vi "Ctrl.StyleFont.vi"(8 "error in (no error)":errorcluster, 10 "Font Info":T1, 11 "Ctl Ref in":refnum<vi>) -> (0 "error out":errorcluster, 3 "Ctl Ref out":refnum<vi>)   [LabVIEW 2017, in "JKI Simple Localization.lvlib"]
uses:
  API/JKI Simple Localization.lvlib
  Definitions/Private/Font Info -- Cluster.ctl
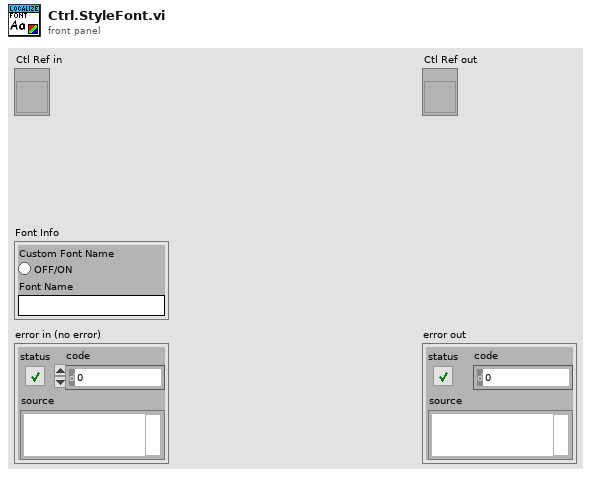
[diagram p1: front panel]
types:
  T1 = typedef "JKI Simple Localization.lvlib/Font Info -- Cluster.ctl" = cluster{"Custom Font Name":bool, "Font Name":string}
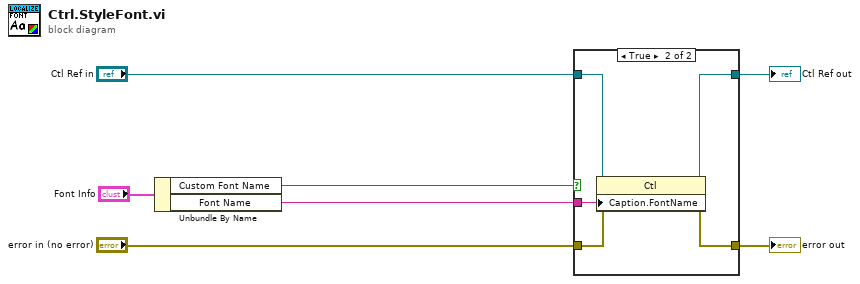
[diagram p0: block diagram]
diagram:
  n1 = Unbundle By Name("Font Info") -> ("Custom Font Name"=w4:bool, "Font Name"=w5:string)
  n2 = case shown="True" w4 {
    tunnel: "error in (no error)" -> [w8 w14]
    tunnel: [w9 w12] -> w2
    tunnel: "Ctl Ref in" -> [w9 w13]
    tunnel: w5 -> [_ w11]
    tunnel: [w8 w10] -> w1
    frame False {
    }
    frame True {
      n3 = property class="Ctl"(reference=w13, error in=w14, "Caption.FontName"=w11) -> (reference out=w12:refnum<vi>, error out=w10:errorcluster)
    }
  }
  "Ctl Ref out" <- w2
  "error out" <- w1
